vi "Close.vi"(8 "error in (no error)":errorcluster caption="entrée d'erreur (pas d'erreur)", 11 "Class Camera IV3-500CA (Default) en entrée":refnum<class "Class Camera IV3-500CA.lvclass">) -> (0 "error out":errorcluster caption="sortie d'erreur", 3 "Class Camera IV3-500CA (Default) en Sortie":refnum<class "Class Camera IV3-500CA.lvclass">)   [LabVIEW 2020, in "Library Instrument & Equipement.lvlib" / "Library Camera.lvlib" / "Class Camera IV3-500CA.lvclass"]
uses:
  Class Camera IV3-500CA.lvclass
  Class Camera IV3-500CA.lvclass/Class Camera IV3-500CA.ctl
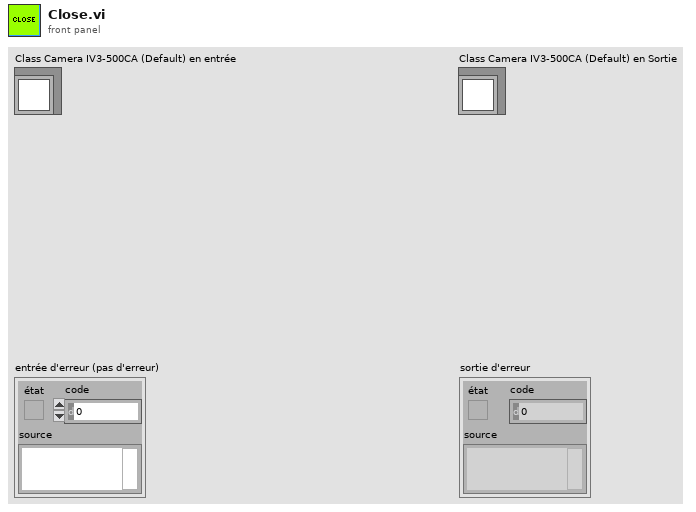
[diagram p1: front panel]
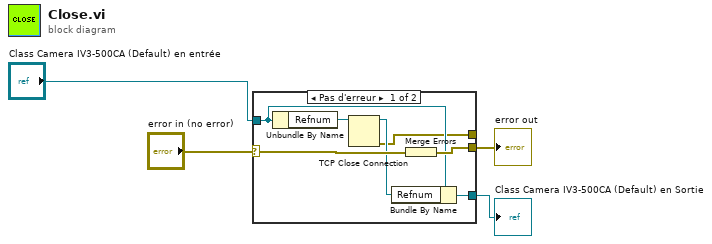
[diagram p0: block diagram]
diagram:
  n1 = case shown="Pas d'erreur" "error in (no error)" {
    selector: "error in (no error)" -> [w10 w13]
    tunnel: [w9 w13] -> w3
    tunnel: [w6 w12] -> w1
    tunnel: "Class Camera IV3-500CA (Default) en entrée" -> [w7 w12]
    tunnel: [w5 _] -> _
    frame No Error {
      n2 = Unbundle By Name(w7) -> ("Refnum"=w11:refnum<k5>)
      n3 = TCP Close Connection(connection ID=w11) -> (connection ID out=w8:refnum<k5>, error out=w5:errorcluster)  [unwired: 2 in]
      n4 = Bundle By Name(cluster=w7, "Refnum"=w8) -> (w6:refnum<class "Class Camera IV3-500CA.lvclass">)
      n5 = Merge Errors(w10) -> (w9:errorcluster)
    }
    frame Error {
    }
  }
  "error out" <- w3
  "Class Camera IV3-500CA (Default) en Sortie" <- w1
